vi "Merged_Voltage.vi"() -> ()   [LabVIEW 2017, in "Examples.lvlib"]
uses:
  Examples.lvlib
panel:
  out "Waveform Chart":dynamicdata(graph)
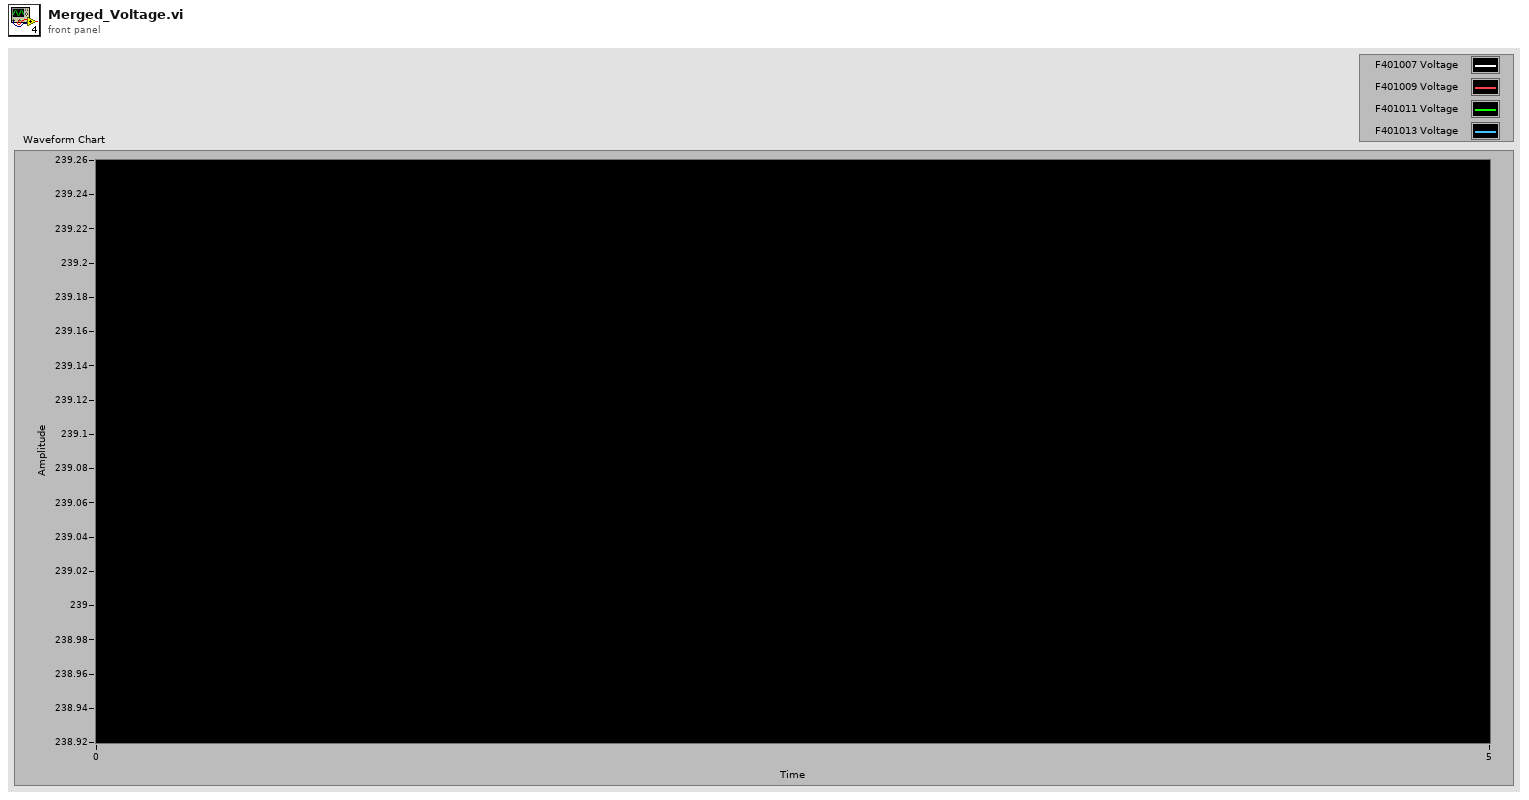
[diagram p1: front panel]
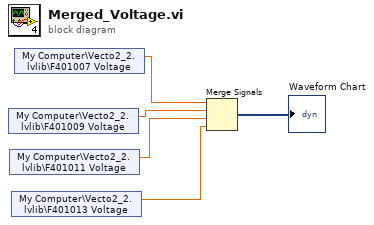
[diagram p0: block diagram]
diagram:
  n1 = shared-variable "My Computer\\Vecto2_2.lvlib\\F401009 Voltage"() -> (w4:sgl)  [unwired: 1 in, 1 out]
  n2 = shared-variable "My Computer\\Vecto2_2.lvlib\\F401011 Voltage"() -> (w3:sgl)  [unwired: 1 in, 1 out]
  n3 = shared-variable "My Computer\\Vecto2_2.lvlib\\F401013 Voltage"() -> (w2:sgl)  [unwired: 1 in, 1 out]
  n4 = shared-variable "My Computer\\Vecto2_2.lvlib\\F401007 Voltage"() -> (w5:sgl)  [unwired: 1 in, 1 out]
  n5 = Merge Signals(w5, w4, w3, w2) -> (→"Waveform Chart":dynamicdata)
